vi "Scan id.vi"() -> (1 "Abort?":bool, 3 "out":string)   [LabVIEW 2021]
panel:
  in  "MSG":string caption="Escriba/Escanee ID Part"
  in  "Title":string
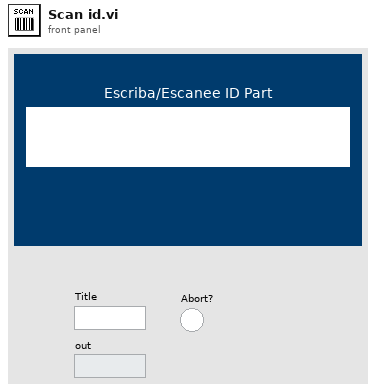
[diagram p1: front panel]
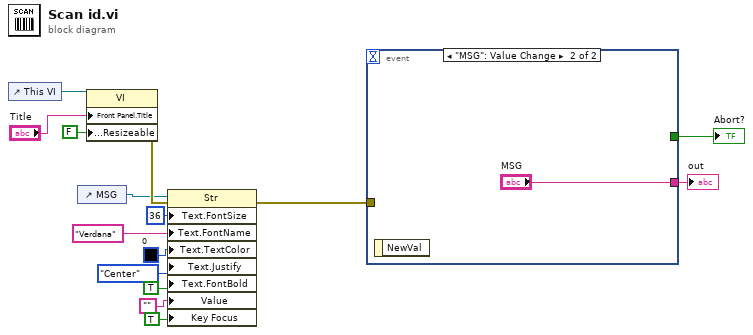
[diagram p0: block diagram]
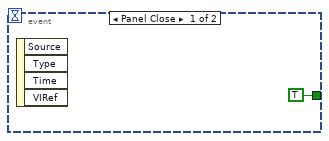
[diagram p2: hidden frame]
diagram:
  n1 = control-ref of="This VI"() -> (w11:refnum<vi>)
  n2 = control-ref of="MSG"() -> (w5:refnum<vi>)
  n3 = property class="VI"(reference=w11, "Front Panel.Title"="Title", "Front Panel.Resizeable"=FALSE ("Front Panel Window:Resizable")) -> (error out=w9:errorcluster)  [unwired: 1 in, 1 out]
  n4 = property on="Property Node" class="Str"(reference=w5, error in=w9, "Text.FontSize"=u32 36 ("Text.Font:Size"), "Text.FontName"="Verdana" ("Text.Font:Name"), "Text.TextColor"=u32 0 ("Text.Text Colors:Text Color"), "Text.Justify"=enum16{"Left", "Center", "Right"}."Center" ("Text.Justification"), "Text.FontBold"=TRUE ("Text.Font:Bold"), "Value"="", "Key Focus"=TRUE) -> (error out=w6:errorcluster)  [unwired: 1 out]
  n5 = event shown="[1] \"MSG\": Value Change" {
    selector: _ -> [_ _]
    dyn-events: _ -> [_ _]
    timeout: _ -> [_ _]
    tunnel: [TRUE _] -> w12
    tunnel: w6 -> [_ _]
    tunnel: [_ "MSG"] -> w2
    event Panel Close {
      n6 = event-data() -> ()  [unwired: 5 out]
    }
    event "MSG": Value Change {
      n7 = event-data() -> ()  [unwired: 2 out]
    }
  }
  "Abort?" <- w12
  "out" <- w2
